vi "FindInstruments.vi"(8 "error in (no error)":errorcluster, 11 "Inovance_Camera in":refnum<class "Inovance_Camera.lvclass">) -> (0 "error out":errorcluster, 3 "Inovance_Camera out":refnum<class "Inovance_Camera.lvclass">)   [LabVIEW 2023, in "Inovance_Camera.lvlib" / "Inovance_Camera.lvclass"]
uses:
  Inovance_Camera.lvclass
  Inovance_Camera.lvclass/Inovance_Camera.ctl
  <vilib>/vision/driver/NI_Vision_Acquisition_Software.lvlib
  Interfaces/InitDeinitInterface/InitDeinitComm Messages/FoundInstruments Msg/FoundInstruments Msg.lvclass
  <vilib>/ActorFramework/Actor/Actor.lvclass
  C:/Program Files/National Instruments/LabVIEW 2023/vi.lib/ActorFramework/Actor/Actor.lvclass
  C:/Users/quantum/Documents/LVDAQ/ConcreteClasses/ConcreteInstrumentClasses/CameraClasses/Inovance_LV/Inovance_Camera/Inovance_Camera.lvclass
  C:/Users/quantum/Documents/LVDAQ/Interfaces/AbstractInstrumentClasses/Cameras_LV/CameraInterface/CameraInterface.lvclass
  C:/Users/quantum/Documents/LVDAQ/Interfaces/InitDeinitInterface/InitDeinit/InitDeinit.lvclass
panel:
  in  "Instruments Found":T1
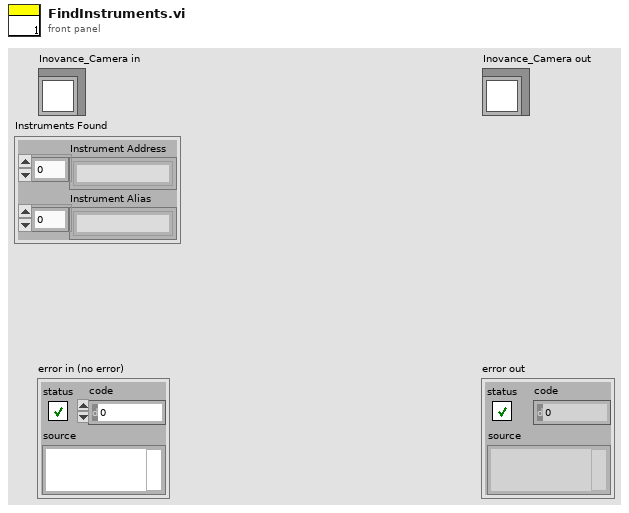
[diagram p1: front panel]
types:
  T1 = cluster{"Instrument Address":string[], "Instrument Alias":string[]}
  T2 = cluster{"Type":u32, "Version":u32, "Flags":u32, "SerialNumberHigh":u32, "SerialNumberLow":u32, "BusType":u32, "InterfaceName":string, "VendorName":string, "ModelName":string, "CameraFileName":string, "CameraAttributeURL":string}[]
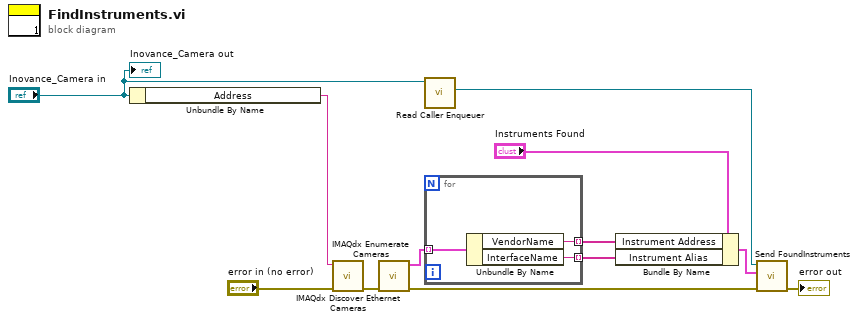
[diagram p0: block diagram]
diagram:
  n1 = Unbundle By Name("Inovance_Camera in") -> ("Address"=w10:string)
  n2 = call <vilib>:"IMAQdx Discover Ethernet Cameras.vi"("error in"="error in (no error)", "Address (Broadcast)"=w10) -> ("error out"=w11:errorcluster)  [unwired: 9 in]
  n3 = call <vilib>:"IMAQdx Enumerate Cameras.vi"("error in"=w11) -> ("error out"=w2:errorcluster, "Camera Information Array"=w12:T2)  [unwired: 9 in]
  n4 = call <vilib>:"Read Caller Enqueuer.vi"("Actor"="Inovance_Camera in") -> ("Caller Enqueuer"=w8:refnum<class "Message Enqueuer.lvclass">)  [unwired: 10 in]
  n5 = for {
    tunnel: w12 -> [w15] mode=indexing
    tunnel: [w14] -> w4 mode=indexing
    tunnel: [w13] -> w5 mode=indexing
    n6 = Unbundle By Name(w15) -> ("VendorName"=w13:string, "InterfaceName"=w14:string)
  }
  n7 = Bundle By Name(cluster="Instruments Found", "Instrument Address"=w5, "Instrument Alias"=w4) -> (w3:T1)
  n8 = call "Send FoundInstruments.vi"("error in (no error)"=w2, "Instruments Found"=w3, "Message Enqueuer"=w8) -> ("error out"=→"error out":errorcluster)  [unwired: 7 in, 1 out]
  "Inovance_Camera out" <- "Inovance_Camera in"
